vi "Lab 1 Exercicio 2.vi"() -> ()   [LabVIEW 2020]
uses:
  <vilib>/MakerHub/LINX/Public/Peripherals/Analog/Analog Read N Chans.vi
  <vilib>/MakerHub/LINX/Public/Peripherals/Digital/Digital Write N Chans.vi
  <vilib>/MakerHub/LINX/Private/Local IO/LinxAnalogRead.vi
  <vilib>/MakerHub/LINX/Public/Utilities/Check Channel.vi
  <vilib>/MakerHub/LINX/Private/Local IO/LinxDigitalWrite.vi
  <vilib>/MakerHub/LINX/Public/Utilities/Open Serial.vi
  <vilib>/MakerHub/LINX/Private/Utilties/Generate Error.vi
  <vilib>/MakerHub/LINX/LMH-LINX.lvlib
panel:
  in  "Digital Output Channel":u8[](array[knob]) scale=0.0..13.0
  in  "Min % Light":dbl=100.0 format="%#_13g"
  in  "Max % Light":dbl=100.0 format="%#_13g"
  out "Light Alarm":bool
  in  "Min ºC Level":dbl=100.0 format="%#_13g"
  in  "Max ºC Level":dbl=100.0 format="%#_13g"
  out "Temperature Alarm":bool
  out "Sensor Values":T1 {"Light Intensity" scale=0.0..5.0; "Temperature" scale=0.0..5.0}
  in  "Analog Channels":u8[](array[knob]) scale=0.0..5.0
  out "Loop Rate (Hz)":u32=200
  in  "Stop Button":bool
  in  "Serial Port":refnum<visa-resource-name>="N/A"
  out "Error Out":errorcluster
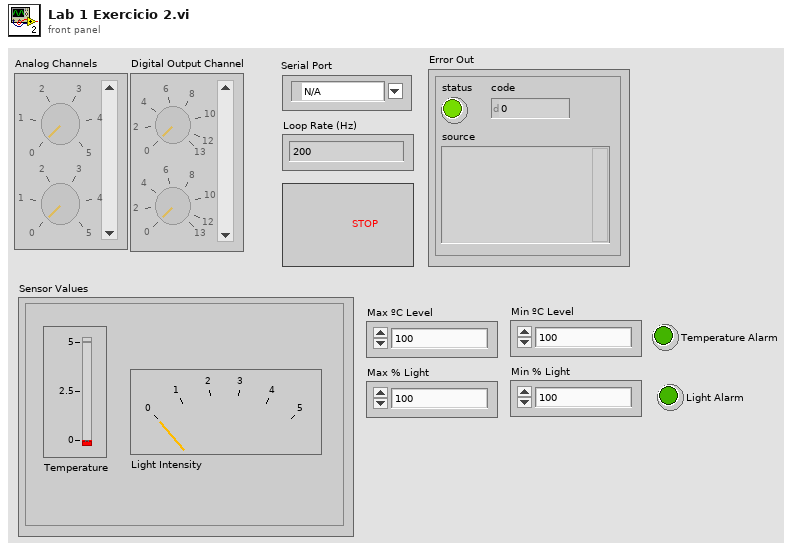
[diagram p1: front panel]
types:
  T1 = cluster{"Temperature":dbl, "Light Intensity":dbl}
  T2 = typedef "LMH-LINX.lvlib/LINX Ref.ctl" = cluster{"IO":T3, "Interface":T4, "LINX Device Config":T5}
  T3 = typedef "LMH-LINX.lvlib/Platform.ctl" = enum16{"Remote", "Local"}
  T4 = typedef "LMH-LINX.lvlib/Interface.ctl" = enum16{"Serial", "TCP"}
  T5 = typedef "LMH-LINX.lvlib/Device.lvlib/LINX Device Config.ctl" = cluster{"Interface":T4, "COM Port":refnum<visa-resource-name>, "TCP Configuration":T6, "Device Family":u8, "Device ID":u8, "Device Name":string, "TCP Ref":refnum<k5>, "Channels":T7}
  T6 = typedef "LMH-LINX.lvlib/Device.lvlib/TCP Config.ctl" = cluster{"IP Address":string, "Port":u16}
  T7 = typedef "LMH-LINX.lvlib/Channels.ctl" = cluster{"DI":u8[], "DO":u8[], "AI":u8[], "AO":u8[], "PWM":u8[], "QE":u8[], "UART":u8[], "I2C 2":u8[], "SPI":u8[], "CAN":u8[], "Servo":u8[], "AI Ref (V)":dbl, "AI Resolution (Bits)":u8, "AO Ref (V)":dbl, "AO Resolution (Bits)":u8}
  T8 = cluster{"Voltages[0]":dbl, "Voltages[1]":dbl, "Voltages[2]":dbl}
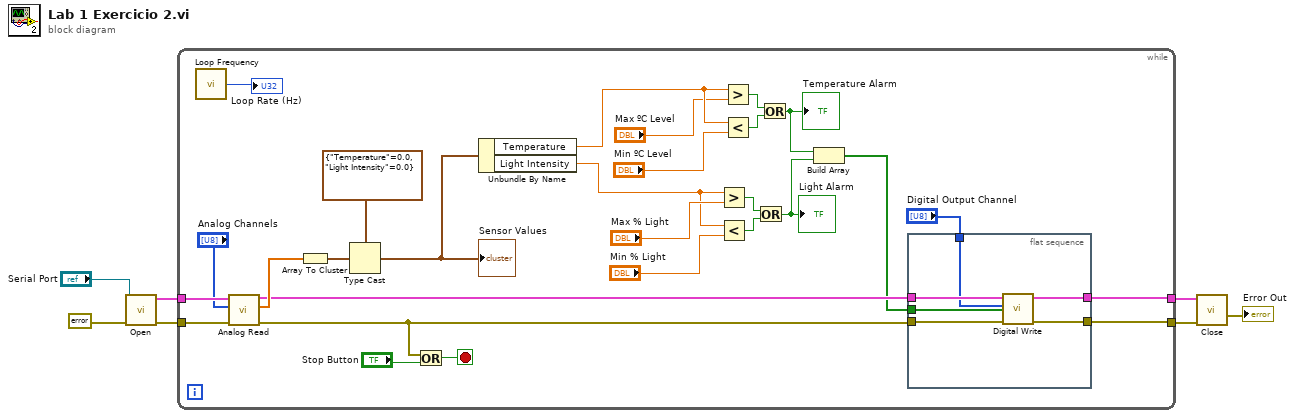
[diagram p0: block diagram]
diagram:
  n1 = call-poly <vilib>:"Open.vi"("Error In"=errorcluster {"status"=FALSE, "code"=0, "source"=""}, "Serial Port"="Serial Port") -> ("Error Out"=w6:errorcluster, "LINX Resource"=w7:T2)  [unwired: 7 in, 1 out]
  n2 = while {
    tunnel: w7 -> [w35]
    tunnel: w6 -> [w34]
    tunnel: [w16] -> w3
    tunnel: [w15] -> w2
    stop <- w33 stop-if-true
    n3 = call <vilib>:"Loop Frequency.vi"() -> ("Loop Rate (Hz)"=→"Loop Rate (Hz)":u32)
    n4 = call-poly <vilib>:"Analog Read.vi"("Error In"=w34, "AI Channel(s)"="Analog Channels", "LINX Resource"=w35) -> ("Error Out"=w13:errorcluster, "Voltages"=w30:dbl[], "LINX Resource"=w14:T2)  [unwired: 5 in, 1 out]
    n5 = Array To Cluster(array=w30) -> (cluster=w29:T8)
    n6 = Type Cast(type=T1 {"Temperature"=0.0, "Light Intensity"=0.0}, x=w29) -> (*(type *) &x=w27:T1)
    "Sensor Values" <- w27
    n7 = Or(x=w13, y="Stop Button") -> (x .or. y?=w33:bool)
    n8 = Unbundle By Name(w27) -> ("Temperature"=w26:dbl, "Light Intensity"=w17:dbl)
    n9 = Greater?(x=w17, y="Max % Light") -> (0:w19:bool)
    n10 = Less?(x=w17, y="Min % Light") -> (x < y?=w20:bool)
    n11 = Greater?(x=w26, y="Max ºC Level") -> (0:w23:bool)
    n12 = Less?(x=w26, y="Min ºC Level") -> (x < y?=w24:bool)
    n13 = Or(x=w19, y=w20) -> (x .or. y?=w10:bool)
    "Light Alarm" <- w10
    n14 = Or(x=w23, y=w24) -> (x .or. y?=w12:bool)
    "Temperature Alarm" <- w12
    n15 = Build Array(w12, w10) -> (w11:bool[])
    n16 = flat-sequence {
      tunnel: w14 -> [w41]
      tunnel: w11 -> [w40]
      tunnel: w13 -> [w39]
      tunnel: [w38] -> w16
      tunnel: [w37] -> w15
      tunnel: "Digital Output Channel" -> [w36]
      frame #0 {
        n17 = call-poly <vilib>:"Digital Write.vi"("Error In"=w39, "Values"=w40, "DO Channels"=w36, "LINX Resource"=w41) -> ("Error Out"=w37:errorcluster, "LINX Resource"=w38:T2)  [unwired: 6 in]
      }
    }
  }
  n18 = call <vilib>:"Close.vi"("Error In"=w2, "LINX Resource"=w3) -> ("Error Out"=→"Error Out":errorcluster)  [unwired: 9 in]
